vi "Finish.vi"   [LabVIEW 2019]
doc: "This VI is called just before exiting. It is expected to close I/O refnum, save collected data, etc."
uses:
  <vilib>/Rock Robotics/WPI/Utilities/WPI_GetSetVariantRefNum.vi
types:
  T1 = typedef "WPI_DigitalInputDevRef.ctl" = cluster{"DevStatus":errorcluster, "DIO Channel":T2}
  T2 = typedef "FPGA_DIOChannel.ctl" = enum8{"DIO 0", "DIO 1", "DIO 2", "DIO 3", "DIO 4", "DIO 5", "DIO 6", "DIO 7", "DIO 8", "DIO 9", "DIO MXP 0", "DIO MXP 1", "DIO MXP 2", "DIO MXP 3", "DIO MXP 4", "DIO MXP 5", "DIO MXP 6", "DIO MXP 7", "DIO MXP 8", "DIO MXP 9", "DIO MXP 10", "DIO MXP 11", "DIO MXP 12", "DIO MXP 13", "DIO MXP 14", "DIO MXP 15", "SPI Port CS1", "SPI Port CS2", "SPI Port CS3", "SPI Port MISO", "SPI Port MOSI", "Invalid"}
  T3 = typedef "WPI_DigitalOutputDevRef.ctl" = cluster{"DIO Channel":T2, "DevStatus":errorcluster}
  T4 = typedef "WPI_JoystickDevRef.ctl" = cluster{"Device":T5}
  T5 = typedef "WPI_JoystickDeviceEnum.ctl" = enum16{"USB 0", "USB 1", "USB 2", "USB 3", "USB 4", "USB 5"}
  T6 = typedef "WPI_SolenoidDevRef.ctl" = cluster{"DevStatus":errorcluster, "Pneumatics Control Module":u8, "Forward Solenoid Channel":T7, "Reverse Solenoid Channel":T7}
  T7 = typedef "WPI_SolenoidChannel.ctl" = enum8{"Solenoid 0", "Solenoid 1", "Solenoid 2", "Solenoid 3", "Solenoid 4", "Solenoid 5", "Solenoid 6", "Solenoid 7", "Invalid"}
  T8 = typedef "WPI_RobotDriveDevRef.ctl" = cluster{"DevStatus":errorcluster, "Motors[]":T9[], "Square Inputs":bool, "Max Output":dbl}
  T9 = typedef "WPI_MotorControlDeviceRef.ctl" = cluster{"DeviceStatus":errorcluster, "Type":T10, "PWM":cluster{"PWM Channel":T11, "DeadBand":T12}, "CAN":cluster{"Device Number":u8, "SetOutput VI Ref":variant, "GetOutput VI Ref":variant, "Enable VI Ref":variant, "Disable VI Ref":variant, "Data":variant}, "Invert":bool, "DIO PWM":cluster{"PWM \"Enable\" Channel":T11, "DIOChannel":T2, "PWM Rate":dbl}}
  T10 = typedef "WPI_MotorControlType.ctl" = enum16{"PWM", "CAN", "DIO PWM"}
  T11 = typedef "FPGA_DIOPWMChannel.ctl" = enum8{"PWM 0", "PWM 1", "PWM 2", "PWM 3", "PWM 4", "PWM 5", "PWM 6", "PWM 7", "PWM 8", "PWM 9", "PWM MXP 0", "PWM MXP 1", "PWM MXP 2", "PWM MXP 3", "PWM MXP 4", "PWM MXP 5", "PWM MXP 6", "PWM MXP 7", "PWM MXP 8", "PWM MXP 9", "Invalid"}
  T12 = typedef "WPI_PWMDeadband.ctl" = cluster{"Name":string, "maxPositivePwm":i32, "minPositivePwm":i32, "centerPwm":i32, "maxNegativePwm":i32, "minNegativePwm":i32, "angularRange":u16}
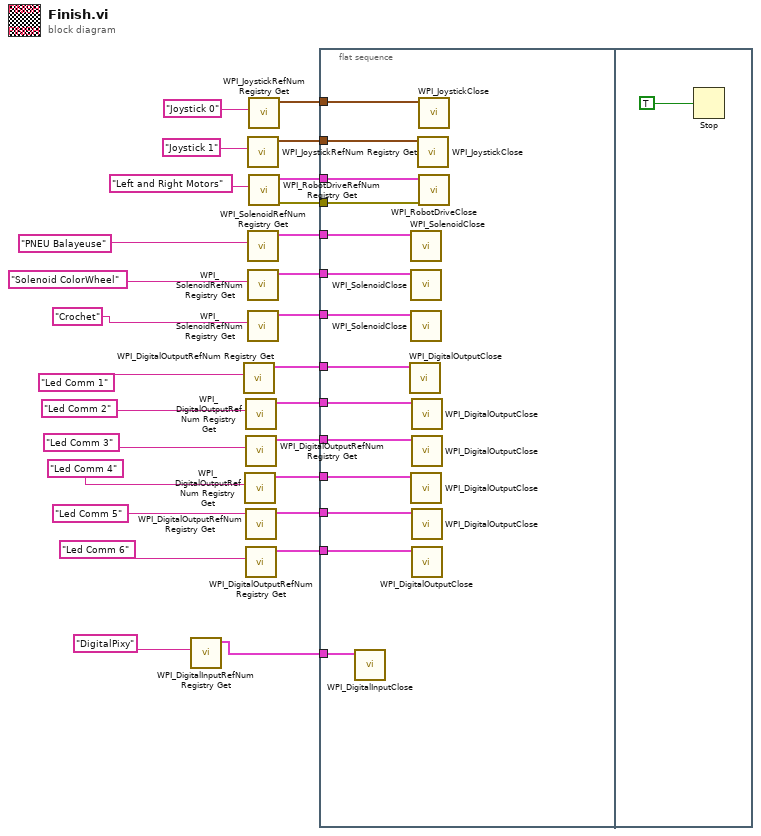
[diagram p0: block diagram]
diagram:
  n1 = call <vilib>:"WPI_DigitalInputRefNum Registry Get.vi"("refnum name"="DigitalPixy") -> ("DigitalInputDevRef"=w14:T1)  [unwired: 9 in, 1 out]
  n2 = call <vilib>:"WPI_DigitalOutputRefNum Registry Get.vi"("refnum name"="Led Comm 1") -> ("DigitalOutputDevRef"=w13:T3)  [unwired: 9 in, 1 out]
  n3 = call <vilib>:"WPI_DigitalOutputRefNum Registry Get.vi"("refnum name"="Led Comm 4") -> ("DigitalOutputDevRef"=w10:T3)  [unwired: 9 in, 1 out]
  n4 = call <vilib>:"WPI_DigitalOutputRefNum Registry Get.vi"("refnum name"="Led Comm 2") -> ("DigitalOutputDevRef"=w12:T3)  [unwired: 9 in, 1 out]
  n5 = call <vilib>:"WPI_DigitalOutputRefNum Registry Get.vi"("refnum name"="Led Comm 3") -> ("DigitalOutputDevRef"=w11:T3)  [unwired: 9 in, 1 out]
  n6 = call <vilib>:"WPI_DigitalOutputRefNum Registry Get.vi"("refnum name"="Led Comm 5") -> ("DigitalOutputDevRef"=w9:T3)  [unwired: 9 in, 1 out]
  n7 = call <vilib>:"WPI_DigitalOutputRefNum Registry Get.vi"("refnum name"="Led Comm 6") -> ("DigitalOutputDevRef"=w8:T3)  [unwired: 9 in, 1 out]
  n8 = call <vilib>:"WPI_JoystickRefNum Registry Get.vi"("refnum name"="Joystick 1") -> ("JoystickDevRef"=w22:T4)  [unwired: 1 in, 9 out]
  n9 = call <vilib>:"WPI_SolenoidRefNum Registry Get.vi"("refnum name"="PNEU Balayeuse") -> ("SolenoidDevRef"=w20:T6)  [unwired: 9 in, 1 out]
  n10 = call <vilib>:"WPI_SolenoidRefNum Registry Get.vi"("refnum name"="Solenoid ColorWheel") -> ("SolenoidDevRef"=w19:T6)  [unwired: 9 in, 1 out]
  n11 = call <vilib>:"WPI_SolenoidRefNum Registry Get.vi"("refnum name"="Crochet") -> ("SolenoidDevRef"=w18:T6)  [unwired: 9 in, 1 out]
  n12 = call <vilib>:"WPI_JoystickRefNum Registry Get.vi"("refnum name"="Joystick 0") -> ("JoystickDevRef"=w24:T4)  [unwired: 1 in, 9 out]
  n13 = call <vilib>:"WPI_RobotDriveRefNum Registry Get.vi"("refnum name"="Left and Right Motors") -> ("error out"=w23:errorcluster, "RobotDriveDevRef"=w25:T8)  [unwired: 1 in, 8 out]
  n14 = flat-sequence {
    tunnel: w25 -> [w41]
    tunnel: w24 -> [w40]
    tunnel: w23 -> [w39]
    tunnel: w22 -> [w38]
    tunnel: w20 -> [w37]
    tunnel: w19 -> [w36]
    tunnel: w18 -> [w35]
    tunnel: w14 -> [w34]
    tunnel: w13 -> [w33]
    tunnel: w12 -> [w32]
    tunnel: w11 -> [w31]
    tunnel: w10 -> [w30]
    tunnel: w9 -> [w29]
    tunnel: w8 -> [w28]
    frame #0 {
      n15 = call <vilib>:"WPI_DigitalInputClose.vi"("DigitalInputDevRef"=w34) -> ()  [unwired: 10 in, 1 out]
      n16 = call <vilib>:"WPI_DigitalOutputClose.vi"("DigitalOutputDevRef"=w33) -> ()  [unwired: 10 in, 1 out]
      n17 = call <vilib>:"WPI_SolenoidClose.vi"("SolenoidDevRef"=w37) -> ()  [unwired: 10 in, 1 out]
      n18 = call <vilib>:"WPI_SolenoidClose.vi"("SolenoidDevRef"=w36) -> ()  [unwired: 10 in, 1 out]
      n19 = call <vilib>:"WPI_SolenoidClose.vi"("SolenoidDevRef"=w35) -> ()  [unwired: 10 in, 1 out]
      n20 = call <vilib>:"WPI_DigitalOutputClose.vi"("DigitalOutputDevRef"=w30) -> ()  [unwired: 10 in, 1 out]
      n21 = call <vilib>:"WPI_DigitalOutputClose.vi"("DigitalOutputDevRef"=w32) -> ()  [unwired: 10 in, 1 out]
      n22 = call <vilib>:"WPI_DigitalOutputClose.vi"("DigitalOutputDevRef"=w31) -> ()  [unwired: 10 in, 1 out]
      n23 = call <vilib>:"WPI_DigitalOutputClose.vi"("DigitalOutputDevRef"=w29) -> ()  [unwired: 10 in, 1 out]
      n24 = call <vilib>:"WPI_DigitalOutputClose.vi"("DigitalOutputDevRef"=w28) -> ()  [unwired: 10 in, 1 out]
      n25 = call <vilib>:"WPI_JoystickClose.vi"("JoystickDevRef"=w38) -> ()  [unwired: 11 out]
      n26 = call <vilib>:"WPI_JoystickClose.vi"("JoystickDevRef"=w40) -> ()  [unwired: 11 out]
      n27 = call <vilib>:"WPI_RobotDriveClose.vi"("error in (no error)"=w39, "RobotDriveDevRef"=w41) -> ()  [unwired: 10 out]
    }
    frame #1 {
      n28 = Stop(stop? (T)=TRUE ("Quit")) -> ()
    }
  }
